vi "Test AO Configuration.vi"(8 "error in (no error)":errorcluster, 11 "Instrument.Lockin in":refnum<class "Instrument.Lockin.lvclass">) -> (0 "error out":errorcluster, 3 "Instrument.Lockin out":refnum<class "Instrument.Lockin.lvclass">)   [LabVIEW 2016]
uses:
  src/Instrument.Lockin/Instrument.Lockin.lvclass
  src/Instrument.Lockin/Typedefs/AO-cluster.ctl
  src/Instrument.Lockin/Typedefs/AO_Amp-array.ctl
  src/Instrument.Lockin/Typedefs/AO_DC-array.ctl
  src/Instrument.Lockin/Typedefs/AO_f-array.ctl
  src/Instrument.Lockin/Typedefs/AO_phi-array.ctl
  src/Instrument.Lockin/Typedefs/Function-array.ctl
  src/Instrument.Lockin/Typedefs/Function-enum.ctl
  <vilib>/addons/_JKI Toolkits/Caraya/classes/Assert/Assert Equal Value and Type_Variant.vi
  <userlib>/_OpenG.lib/numeric/numeric.llb/Random Number Within Range - I32__ogtk.vi
  <userlib>/_OpenG.lib/numeric/numeric.llb/Random Number Within Range - DBL__ogtk.vi
  <vilib>/addons/_JKI Toolkits/Caraya/classes/Assert/Assert Almost Equal_Float.vi
  <vilib>/addons/_JKI Toolkits/Caraya/classes/Assert/Assert Equal Value_Variant.vi
  <vilib>/addons/_JKI Toolkits/Caraya/classes/Test/Test.lvclass
  <vilib>/addons/_JKI Toolkits/Caraya/classes/Assert/Assert.lvclass
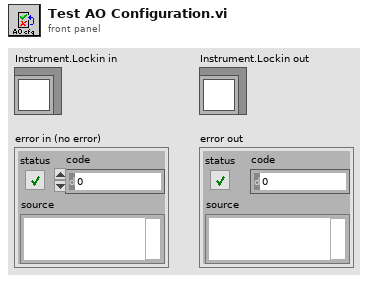
[diagram p1: front panel]
types:
  T1 = typedef "Instrument.Lockin.lvclass/AO-cluster.ctl" = cluster{"AO Amp (V)":T2, "AO DC (V)":T3, "AO f (Hz)":T4, "AO Phase (°)":T5, "Function":T6, "I+":bool[], "Sweeping":bool[]}
  T2 = typedef "Instrument.Lockin.lvclass/AO_Amp-array.ctl" = dbl[]
  T3 = typedef "Instrument.Lockin.lvclass/AO_DC-array.ctl" = dbl[]
  T4 = typedef "Instrument.Lockin.lvclass/AO_f-array.ctl" = dbl[]
  T5 = typedef "Instrument.Lockin.lvclass/AO_phi-array.ctl" = dbl[]
  T6 = typedef "Instrument.Lockin.lvclass/Function-array.ctl" = T7[]
  T7 = typedef "Instrument.Lockin.lvclass/Function-enum.ctl" = enum16{"Sine", "Triangle", "Square", "Sawtooth"}
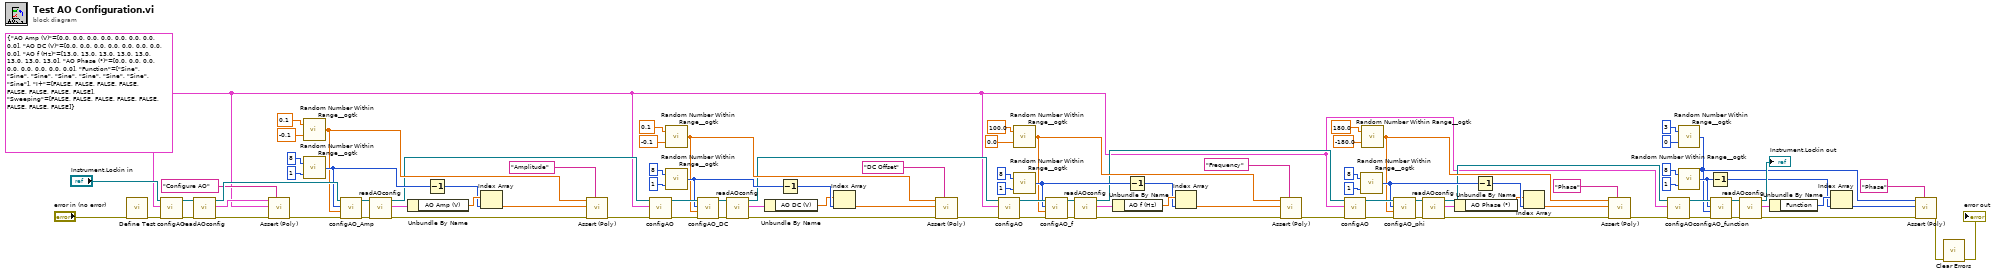
[diagram p0: block diagram]
diagram:
  w3 = T1 {"AO Amp (V)"=[0.0, 0.0, 0.0, 0.0, 0.0, 0.0, 0.0, 0.0], "AO DC (V)"=[0.0, 0.0, 0.0, 0.0, 0.0, 0.0, 0.0, 0.0], "AO f (Hz)"=[13.0, 13.0, 13.0, 13.0, 13.0, 13.0, 13.0, 13.0], "AO Phase (°)"=[0.0, 0.0, 0.0, 0.0, 0.0, 0.0, 0.0, 0.0], "Function"=[enum."Sine", enum."Sine", enum."Sine", enum."Sine", enum."Sine", enum."Sine", enum."Sine", enum."Sine"], "I+"=[FALSE, FALSE, FALSE, FALSE, FALSE, FALSE, FALSE, FALSE], "Sweeping"=[FALSE, FALSE, FALSE, FALSE, FALSE, FALSE, FALSE, FALSE]} ("Channels: AO")
  n1 = call <vilib>:"Define Test.vi"("error in (no error)"="error in (no error)") -> ("error out"=w84:errorcluster)  [unwired: 10 in]
  n2 = call "configAO.vi"("error in (no error)"=w84, "Channels: AO"=w3, "Instrument.Lockin in"="Instrument.Lockin in") -> ("error out"=w88:errorcluster, "Instrument.Lockin out"=w87:refnum<class "Instrument.Lockin.lvclass">)  [unwired: 7 in]
  n3 = call "readAOconfig.vi"("error in (no error)"=w88, "Instrument.Lockin in"=w87) -> ("error out"=w81:errorcluster, "AOconfig"=w83:T1, "Instrument.Lockin out"=w89:refnum<class "Instrument.Lockin.lvclass">)  [unwired: 7 in]
  n4 = call-poly <vilib>:"Assert (Poly).vi"("Label"="Configure AO", "error in (no error)"=w81, "Y"=w3, "X"=w83) -> ("error out"=w80:errorcluster)  [unwired: 7 in]
  n5 = call-poly <userlib>:"Random Number Within Range__ogtk.vi"("High"=0.1, "Low"=-0.1) -> ("Random Number"=w71:dbl)  [unwired: 3 in]
  n6 = call-poly <userlib>:"Random Number Within Range__ogtk.vi"("High"=8, "Low"=1) -> ("Random Number"=w75:i32)  [unwired: 3 in]
  n7 = call "configAO_Amp.vi"("error in (no error)"=w80, "Amplitude (V)"=w71, "AO Channel"=w75, "Instrument.Lockin in"=w89) -> ("error out"=w91:errorcluster, "Instrument.Lockin out"=w90:refnum<class "Instrument.Lockin.lvclass">)  [unwired: 6 in]
  n8 = call "readAOconfig.vi"("error in (no error)"=w91, "Instrument.Lockin in"=w90) -> ("error out"=w68:errorcluster, "AOconfig"=w79:T1, "Instrument.Lockin out"=w66:refnum<class "Instrument.Lockin.lvclass">)  [unwired: 7 in]
  n9 = Unbundle By Name(w79) -> ("AO Amp (V)"=w78:T2)
  n10 = Decrement(x=w75) -> (x-1=w77:i32)
  n11 = Index Array(array=w78, index=w77) -> (element=w70:dbl)
  n12 = call-poly <vilib>:"Assert (Poly).vi"("Label"="Amplitude", "error in (no error)"=w68, "Y"=w70, "X"=w71) -> ("error out"=w67:errorcluster)  [unwired: 7 in]
  n13 = call "configAO.vi"("error in (no error)"=w67, "Channels: AO"=w3, "Instrument.Lockin in"=w66) -> ("error out"=w60:errorcluster, "Instrument.Lockin out"=w61:refnum<class "Instrument.Lockin.lvclass">)  [unwired: 7 in]
  n14 = call-poly <userlib>:"Random Number Within Range__ogtk.vi"("High"=0.1, "Low"=-0.1) -> ("Random Number"=w52:dbl)  [unwired: 3 in]
  n15 = call-poly <userlib>:"Random Number Within Range__ogtk.vi"("High"=8, "Low"=1) -> ("Random Number"=w55:i32)  [unwired: 3 in]
  n16 = call "configAO_DC.vi"("error in (no error)"=w60, "DC (V)"=w52, "AO Channel"=w55, "Instrument.Lockin in"=w61) -> ("error out"=w93:errorcluster, "Instrument.Lockin out"=w92:refnum<class "Instrument.Lockin.lvclass">)  [unwired: 6 in]
  n17 = call "readAOconfig.vi"("error in (no error)"=w93, "Instrument.Lockin in"=w92) -> ("error out"=w53:errorcluster, "AOconfig"=w54:T1, "Instrument.Lockin out"=w51:refnum<class "Instrument.Lockin.lvclass">)  [unwired: 7 in]
  n18 = Unbundle By Name(w54) -> ("AO DC (V)"=w56:T3)
  n19 = Decrement(x=w55) -> (x-1=w57:i32)
  n20 = Index Array(array=w56, index=w57) -> (element=w58:dbl)
  n21 = call-poly <vilib>:"Assert (Poly).vi"("Label"="DC Offset", "error in (no error)"=w53, "Y"=w58, "X"=w52) -> ("error out"=w49:errorcluster)  [unwired: 7 in]
  n22 = call "configAO.vi"("error in (no error)"=w49, "Channels: AO"=w3, "Instrument.Lockin in"=w51) -> ("error out"=w48:errorcluster, "Instrument.Lockin out"=w50:refnum<class "Instrument.Lockin.lvclass">)  [unwired: 7 in]
  n23 = call-poly <userlib>:"Random Number Within Range__ogtk.vi"("High"=100.0, "Low"=0.0) -> ("Random Number"=w38:dbl)  [unwired: 3 in]
  n24 = call-poly <userlib>:"Random Number Within Range__ogtk.vi"("High"=8, "Low"=1) -> ("Random Number"=w39:i32)  [unwired: 3 in]
  n25 = call "configAO_f.vi"("error in (no error)"=w48, "Frequency (Hz)"=w38, "AO Channel"=w39, "Instrument.Lockin in"=w50) -> ("error out"=w95:errorcluster, "Instrument.Lockin out"=w94:refnum<class "Instrument.Lockin.lvclass">)  [unwired: 6 in]
  n26 = call "readAOconfig.vi"("error in (no error)"=w95, "Instrument.Lockin in"=w94) -> ("error out"=w36:errorcluster, "AOconfig"=w37:T1, "Instrument.Lockin out"=w34:refnum<class "Instrument.Lockin.lvclass">)  [unwired: 7 in]
  n27 = Unbundle By Name(w37) -> ("AO f (Hz)"=w47:T4)
  n28 = Decrement(x=w39) -> (x-1=w46:i32)
  n29 = Index Array(array=w47, index=w46) -> (element=w45:dbl)
  n30 = call-poly <vilib>:"Assert (Poly).vi"("Label"="Frequency", "error in (no error)"=w36, "Y"=w45, "X"=w38) -> ("error out"=w33:errorcluster)  [unwired: 7 in]
  n31 = call "configAO.vi"("error in (no error)"=w33, "Channels: AO"=w3, "Instrument.Lockin in"=w34) -> ("error out"=w20:errorcluster, "Instrument.Lockin out"=w35:refnum<class "Instrument.Lockin.lvclass">)  [unwired: 7 in]
  n32 = call-poly <userlib>:"Random Number Within Range__ogtk.vi"("High"=8, "Low"=1) -> ("Random Number"=w23:i32)  [unwired: 3 in]
  n33 = call-poly <userlib>:"Random Number Within Range__ogtk.vi"("High"=180.0, "Low"=-180.0) -> ("Random Number"=w22:dbl)  [unwired: 3 in]
  n34 = call "configAO_phi.vi"("error in (no error)"=w20, "Phase (°)"=w22, "AO Channel"=w23, "Instrument.Lockin in"=w35) -> ("error out"=w97:errorcluster, "Instrument.Lockin out"=w96:refnum<class "Instrument.Lockin.lvclass">)  [unwired: 6 in]
  n35 = call "readAOconfig.vi"("error in (no error)"=w97, "Instrument.Lockin in"=w96) -> ("error out"=w21:errorcluster, "AOconfig"=w24:T1, "Instrument.Lockin out"=w18:refnum<class "Instrument.Lockin.lvclass">)  [unwired: 7 in]
  n36 = Unbundle By Name(w24) -> ("AO Phase (°)"=w25:T5)
  n37 = Decrement(x=w23) -> (x-1=w26:i32)
  n38 = Index Array(array=w25, index=w26) -> (element=w27:dbl)
  n39 = call-poly <vilib>:"Assert (Poly).vi"("Label"="Phase", "error in (no error)"=w21, "Y"=w27, "X"=w22) -> ("error out"=w19:errorcluster)  [unwired: 7 in]
  n40 = call "configAO.vi"("error in (no error)"=w19, "Channels: AO"=w3, "Instrument.Lockin in"=w18) -> ("error out"=w16:errorcluster, "Instrument.Lockin out"=w17:refnum<class "Instrument.Lockin.lvclass">)  [unwired: 7 in]
  n41 = call-poly <userlib>:"Random Number Within Range__ogtk.vi"("High"=3, "Low"=0) -> ("Random Number"=w5:i32)  [unwired: 3 in]
  n42 = call-poly <userlib>:"Random Number Within Range__ogtk.vi"("High"=8, "Low"=1) -> ("Random Number"=w8:i32)  [unwired: 3 in]
  n43 = Decrement(x=w8) -> (x-1=w14:i32)
  n44 = call "configAO_function.vi"("error in (no error)"=w16, "Function"=w5, "AO Channel"=w8, "Instrument.Lockin in"=w17) -> ("error out"=w99:errorcluster, "Instrument.Lockin out"=w98:refnum<class "Instrument.Lockin.lvclass">)  [unwired: 6 in]
  n45 = call "readAOconfig.vi"("error in (no error)"=w99, "Instrument.Lockin in"=w98) -> ("error out"=w4:errorcluster, "AOconfig"=w9:T1, "Instrument.Lockin out"=→"Instrument.Lockin out":refnum<class "Instrument.Lockin.lvclass">)  [unwired: 7 in]
  n46 = Unbundle By Name(w9) -> ("Function"=w15:T6)
  n47 = Index Array(array=w15, index=w14) -> (element=w13:T7)
  n48 = call-poly <vilib>:"Assert (Poly).vi"("Label"="Phase", "error in (no error)"=w4, "Y"=w13, "X"=w5) -> ("error out"=w2:errorcluster)  [unwired: 7 in]
  n49 = call <vilib>:"Clear Errors.vi"("error in (no error)"=w2) -> ("error out"=→"error out":errorcluster)  [unwired: 5 in, 1 out]
